vi "Example Graph.vi"() -> ()   [LabVIEW 2013]
uses:
  C:/tf/play/labview/Tinkerforge.dll
  Tinkerforge.dll
panel:
  in  "stop":bool
  out "graph":sgl[](graph)
  in  "uid":string="amb"
  in  "port":i32=4223
  in  "host":string="localhost"
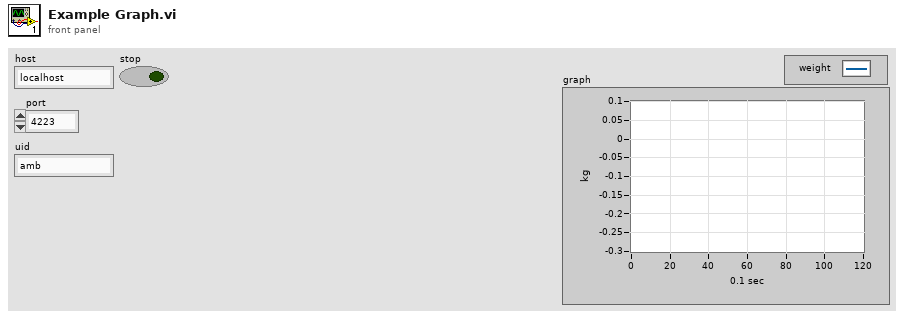
[diagram p1: front panel]
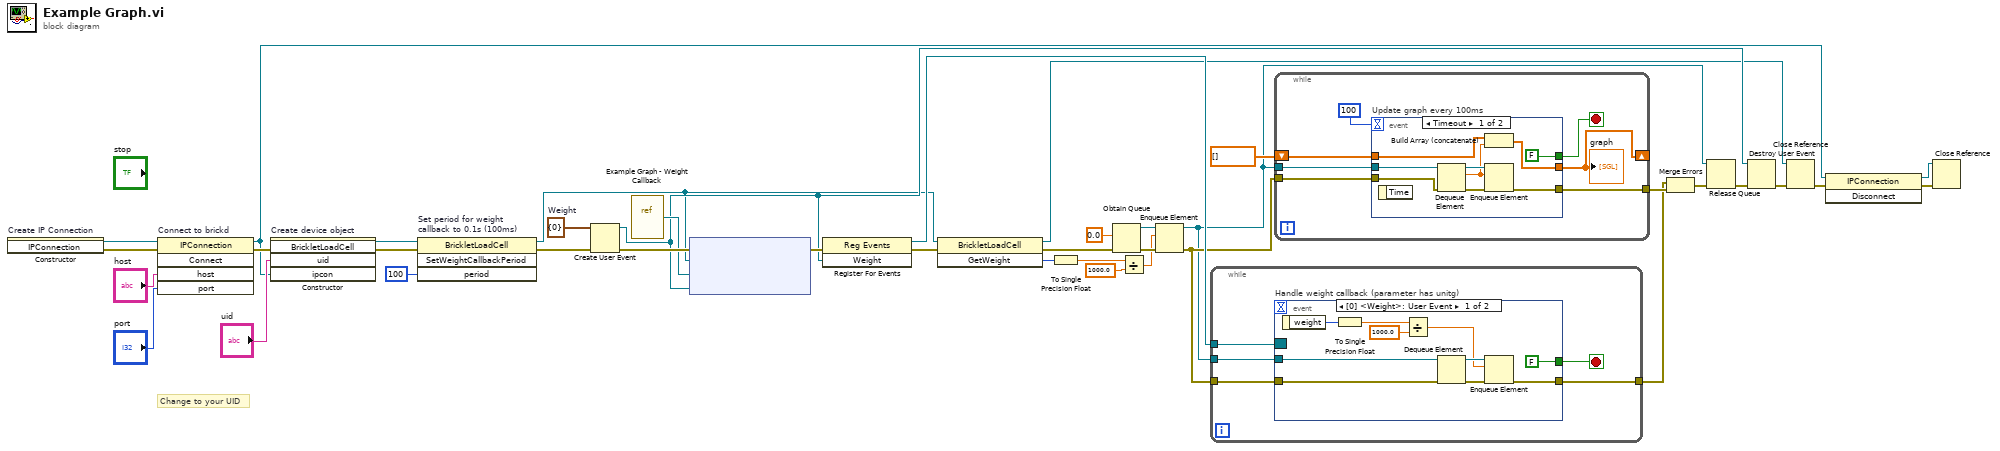
[diagram p0: block diagram]
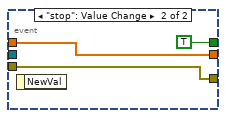
[diagram p2: hidden frame]
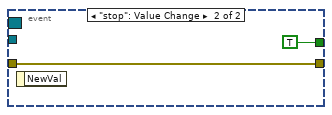
[diagram p3: hidden frame]
diagram:
  w24 = cluster{"weight":i32} {"weight"=0}  # Weight
  # "Change to your UID"
  n1 = constructor on="Create IP Connection" class="IPConnection"() -> (reference out=w39:refnum<k24>, error out=w9:errorcluster)  [unwired: 3 in, 1 out]
  n2 = invoke on="Connect to brickd" class="IPConnection" method="Connect"(reference=w39, error in=w9, "host"="host", "port"="port") -> (reference out=w32:refnum<k24>, error out=w35:errorcluster)  [unwired: 1 in, 3 out]
  n3 = constructor on="Create device object" class="BrickletLoadCell"(error in=w35, "uid"="uid", "ipcon"=w32) -> (reference out=w21:refnum<k24>, error out=w23:errorcluster)  [unwired: 2 in, 3 out]
  n4 = invoke on="Set period for weight\ncallback to 0.1s (100ms)" class="BrickletLoadCell" method="SetWeightCallbackPeriod"(reference=w21, error in=w23, "period"=i64 100) -> (reference out=w6:refnum<k24>, error out=w22:errorcluster)  [unwired: 1 in, 2 out]
  n5 = Create User Event(user event datatype=w24, error in=w22) -> (user event=w26:refnum<user-event>, error out=w30:errorcluster)
  n6 = vi-ref "Example Graph - Weight Callback.vi"() -> ("vi reference"=w28:refnum<vi>)
  n7 = node ("Register Event Callback")(w30, w6, w28, w26) -> (w29:errorcluster)  [unwired: 1 in, 1 out]
  n8 = register-events(error in=w29, w26) -> (reference out=w27:refnum<event-registration>, error out=w8:errorcluster)  [unwired: 1 in]
  n9 = invoke class="BrickletLoadCell" method="GetWeight"(reference=w6, error in=w8) -> (reference out=w5:refnum<k24>, error out=w7:errorcluster, "GetWeight"=w2:i32)  [unwired: 1 in]
  n10 = To Single Precision Float(number=w2) -> (single precision float=w4:sgl)
  n11 = Obtain Queue(element data type=sgl 0.0, error in (no error)=w7) -> (queue out=w13:refnum<queue>, error out=w15:errorcluster)  [unwired: 3 in, 1 out]
  n12 = Divide(x=w4, y=sgl 1000.0) -> (x/y=w1:sgl)
  n13 = Enqueue Element(queue=w13, element=w1, error in (no error)=w15) -> (queue out=w10:refnum<queue>, error out=w14:errorcluster)  [unwired: 1 in, 1 out]
  n14 = while {
    tunnel: w27 -> [w44]
    tunnel: [w42] -> w18
    tunnel: w14 -> [w43]
    tunnel: w10 -> [w41]
    stop <- w40 stop-if-true
    n15 = event "Handle weight callback (parameter has unitg)" shown="[0] <Weight>: User Event" {
      selector: w44 -> [_ _]
      dyn-events: _ -> [_ _]
      timeout: _ -> [_ _]
      tunnel: w43 -> [w51 w55]
      tunnel: [w49 w55] -> w42
      tunnel: w41 -> [w48 _]
      tunnel: [FALSE TRUE] -> w40
      event User Event {
        n16 = event-data() -> ("weight"=w52:i32)  [unwired: 1 in]
        n17 = To Single Precision Float(number=w52) -> (single precision float=w53:sgl)
        n18 = Divide(x=w53, y=sgl 1000.0) -> (x/y=w46:sgl)
        n19 = Dequeue Element(queue=w48, error in (no error)=w51) -> (queue out=w47:refnum<queue>, error out=w50:errorcluster)  [unwired: 1 in, 2 out]
        n20 = Enqueue Element(queue=w47, element=w46, error in (no error)=w50) -> (error out=w49:errorcluster)  [unwired: 1 in, 2 out]
      }
      event "stop": Value Change {
        n21 = event-data() -> ()  [unwired: 1 in, 1 out]
      }
    }
  }
  n22 = while {
    tunnel: [w59] -> w19
    tunnel: w14 -> [w60]
    shift-right: [w61] -> _
    shift-left: sgl[] [] -> [w62]
    tunnel: w10 -> [w58]
    stop <- w57 stop-if-true
    n23 = event "Update graph every 100ms" shown="[0] Timeout" {
      selector: _ -> [_ _]
      dyn-events: _ -> [_ _]
      timeout: 100 -> [_ _]
      tunnel: [w72 w74] -> w61
      tunnel: w62 -> [w65 w74]
      tunnel: w60 -> [w71 w73]
      tunnel: [w68 w73] -> w59
      tunnel: w58 -> [w70 _]
      tunnel: [FALSE TRUE] -> w57
      event Timeout {
        n24 = event-data() -> ()  [unwired: 1 in, 1 out]
        n25 = Dequeue Element(queue=w70, error in (no error)=w71) -> (queue out=w67:refnum<queue>, element=w66:sgl, error out=w69:errorcluster)  [unwired: 1 in, 1 out]
        n26 = Build Array (concatenate)(w65, w66) -> (w72:sgl[])
        n27 = Enqueue Element(queue=w67, element=w66, error in (no error)=w69) -> (error out=w68:errorcluster)  [unwired: 1 in, 2 out]
      }
      event "stop": Value Change {
        n28 = event-data() -> ()  [unwired: 1 in, 1 out]
      }
    }
    "graph" <- w61
  }
  n29 = Merge Errors(w18, w19) -> (w12:errorcluster)
  n30 = Release Queue(queue=w10, error in (no error)=w12) -> (error out=w11:errorcluster)  [unwired: 1 in, 2 out]
  n31 = Destroy User Event(user event=w26, error in=w11) -> (error out=w25:errorcluster)
  n32 = Close Reference(reference=w5, error in (no error)=w25) -> (error out=w34:errorcluster)
  n33 = invoke class="IPConnection" method="Disconnect"(reference=w32, error in=w34) -> (reference out=w31:refnum<k24>, error out=w33:errorcluster)  [unwired: 1 in, 1 out]
  n34 = Close Reference(reference=w31, error in (no error)=w33) -> ()  [unwired: 1 out]
